vi "NHMFL SCM Oxford IPS initialize.vi"(0 "VISA session":refnum<visa-resource-name>="GPIB0::22::INSTR") -> (1 "dup VISA session":refnum<visa-resource-name>, 2 "Output Cluster":T2 {"MaxLambdaCurrent [A]" format="%.2f"; "LambdaRates [A/min]" format="%.5e"; "MaxNormalCurrent [A]" format="%.2f"; "StabilitySetting [%]" format="%.2f"; "FieldCurrentRatio [T/A]" format="%.2f"; "SwitchWaitTime [s]" format="%.2f"; "SwitchHtrCurrent [mA]" format="%.2f"; "TrainRates [A/min]" format="%.5e"; "NormalRates [A/min]" format="%.5e"; "Breakpts [A]" format="%.5e"}, 3 "Mode Out":T1(ring), 4 "Programmed Field":dbl format="%.2f", 5 "Ramp Rate":dbl format="%.2f", 6 "Persistent Field":dbl format="%.2f", 7 "Persistent":bool)   [LabVIEW 2024]
panel:
  in  "Input Cluster":T2 {"MaxLambdaCurrent [A]" format="%.2f"; "LambdaRates [A/min]" format="%.5e"; "MaxNormalCurrent [A]" format="%.2f"; "StabilitySetting [%]" format="%.2f"; "FieldCurrentRatio [T/A]" format="%.2f"; "SwitchWaitTime [s]" format="%.2f"; "SwitchHtrCurrent [mA]" format="%.2f"; "TrainRates [A/min]" format="%.5e"; "NormalRates [A/min]" format="%.5e"; "Breakpts [A]" format="%.5e"}
  out "Field":dbl format="%.2f"
  out "error out":errorcluster
  in  "error in (no error)":errorcluster
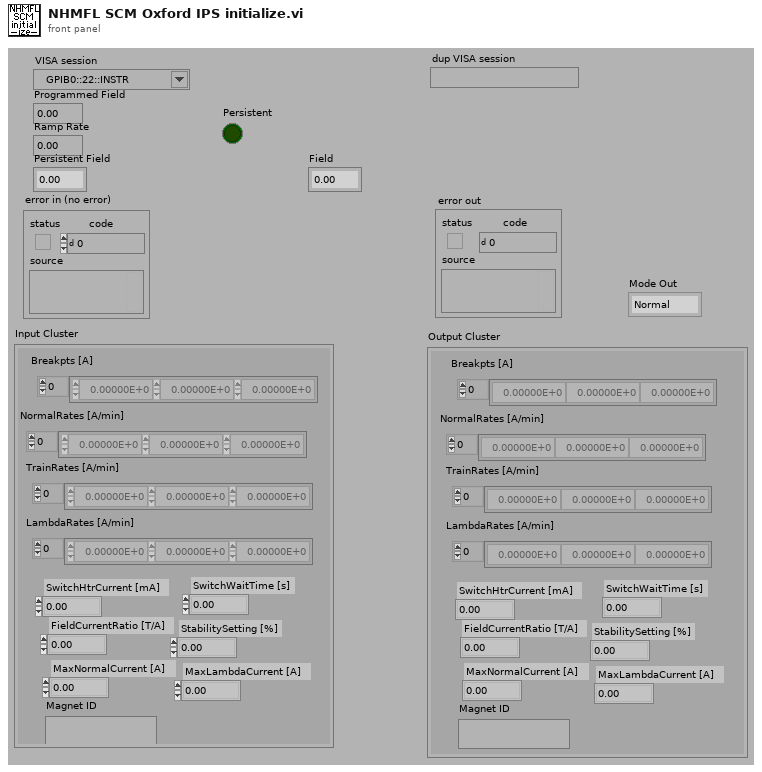
[diagram p1: front panel]
types:
  T1 = enum16{"Normal", "Train", "Lambda", "Train & Lambda"}
  T2 = cluster{"Breakpts [A]":dbl[], "NormalRates [A/min]":dbl[], "TrainRates [A/min]":dbl[], "SwitchHtrCurrent [mA]":dbl, "SwitchWaitTime [s]":dbl, "FieldCurrentRatio [T/A]":dbl, "StabilitySetting [%]":dbl, "MaxNormalCurrent [A]":dbl, "Magnet ID":string, "LambdaRates [A/min]":dbl[], "MaxLambdaCurrent [A]":dbl}
  T3 = enum16{"No Response", "Ramping to programmed field ", "Holding at programmed field", "Paused", "Ramp Manual Up", "Ramp Manual Down", "Ramping to Zero", "QUENCH", "Heating Persistence Switch", "At Zero Current"}
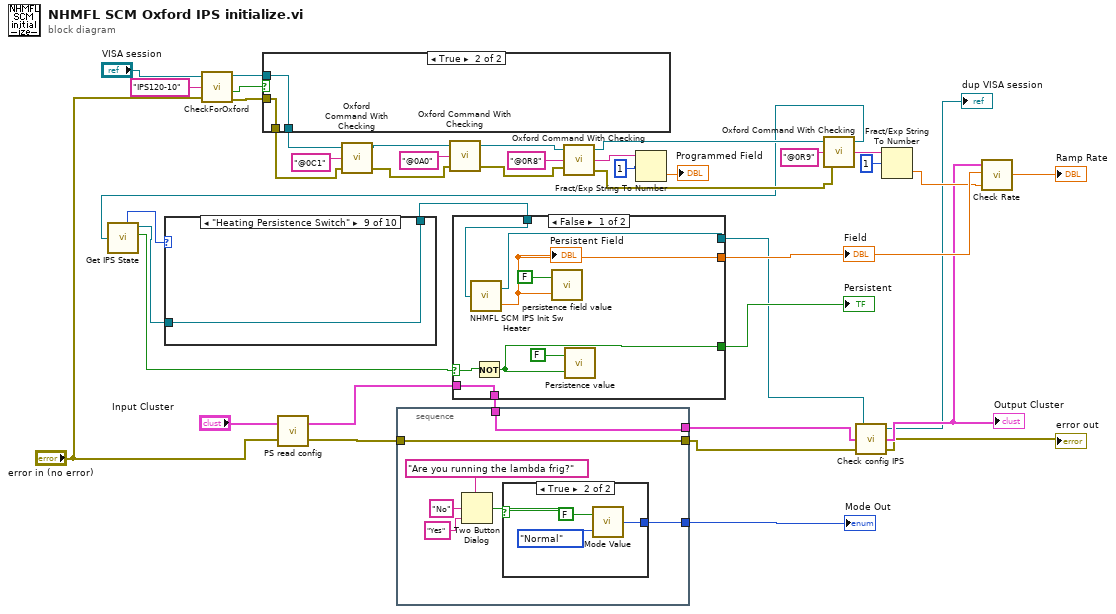
[diagram p0: block diagram]
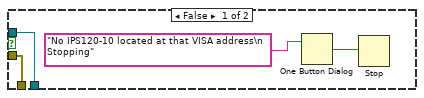
[diagram p2: hidden frame]
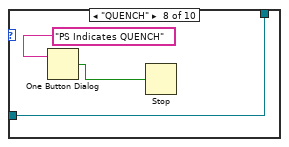
[diagram p10: hidden frame]
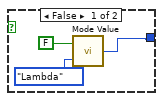
[diagram p12: hidden frame]
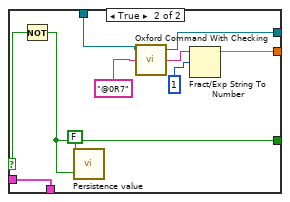
[diagram p13: hidden frame]
diagram:
  n1 = call "CheckForOxford.vi"("VISA session"="VISA session", "search string"="IPS120-10", "error in (no error)"="error in (no error)") -> ("dup VISA session"=w29:refnum<visa-resource-name>, "Instrument detected"=w31:bool, "error out"=w30:errorcluster)  [unwired: 1 out]
  n2 = case shown="True" w31 {
    tunnel: [w45 w49] -> w27
    tunnel: w30 -> [w45 w49]
    tunnel: [w44 w48] -> w16
    tunnel: w29 -> [w44 w48]
    frame False {
      n3 = One Button Dialog(message="No IPS120-10 located at that VISA address\n                                 Stopping") -> (true=w46:bool)  [unwired: 1 in]
      n4 = Stop(stop? (T)=w46) -> ()
    }
    frame True {
    }
  }
  n5 = call "PS read config.vi"("error in (no error)"="error in (no error)", "Input Cluster"="Input Cluster") -> ("error out"=w39:errorcluster, "output cluster"=w38:T2)
  n6 = call "Oxford Command With Checking.vi"("error in (no error)"=w27, "Command"="@0C1" ("Command String"), "VISA session"=w16) -> ("error out"=w7:errorcluster, "dup VISA session"=w8:refnum<visa-resource-name>)  [unwired: 1 out]
  n7 = call "Oxford Command With Checking.vi"("error in (no error)"=w7, "Command"="@0A0" ("Command String"), "VISA session"=w8) -> ("error out"=w6:errorcluster, "dup VISA session"=w5:refnum<visa-resource-name>)  [unwired: 1 out]
  n8 = call "Oxford Command With Checking.vi"("error in (no error)"=w6, "Command"="@0R8" ("Command String"), "VISA session"=w5) -> ("error out"=w19:errorcluster, "String Read"=w26:string, "dup VISA session"=w25:refnum<visa-resource-name>)
  n9 = Fract/Exp String To Number(string=w26, offset=1) -> (number=→"Programmed Field":dbl)  [unwired: 2 in, 1 out]
  n10 = call "Oxford Command With Checking.vi"("error in (no error)"=w19, "Command"="@0R9" ("Command String"), "VISA session"=w25) -> ("String Read"=w23:string, "dup VISA session"=w1:refnum<visa-resource-name>)  [unwired: 1 out]
  n11 = call "Get IPS State.vi"("VISA session"=w1) -> ("State"=w18:T3, "dup VISA session"=w3:refnum<visa-resource-name>, "Switch Heater"=w17:bool)  [unwired: 1 in, 2 out]
  n12 = case shown="\"Heating Persistence Switch\"" w18 {
    tunnel: [w50 w51 w52 w53 w54 w55 w56 w57 w60 w61] -> w35
    tunnel: w3 -> [w50 w51 w52 w53 w54 w55 w56 w57 w60 w61]
    frame "No Response", Default {
    }
    frame "Holding at programmed field" {
    }
    frame "Ramping to programmed field " {
    }
    frame "Paused" {
    }
    frame "Ramp Manual Up" {
    }
    frame "Ramp Manual Down" {
    }
    frame "Ramping to Zero" {
    }
    frame "QUENCH" {
      n13 = One Button Dialog(message="PS Indicates QUENCH") -> (true=w58:bool)  [unwired: 1 in]
      n14 = Stop(stop? (T)=w58) -> ()
    }
    frame "Heating Persistence Switch" {
    }
    frame "At Zero Current" {
    }
  }
  n15 = case shown="False" w17 {
    selector: w17 -> [w67 w78]
    tunnel: [w66 w77] -> w43
    tunnel: w35 -> [w64 w74]
    tunnel: [w63 w76] -> w40
    tunnel: w38 -> [w65 w75]
    tunnel: [w65 w75] -> w37
    tunnel: [w62 w73] -> w11
    frame False {
      n16 = call "NHMFL SCM IPS Init Sw Heater.vi"("VISA session"=w64) -> ("dup VISA session"=w62:refnum<visa-resource-name>, "Persistent Field"=w63:dbl)
      "Persistent Field" <- w63
      n17 = Not(x=w67) -> (.not. x?=w66:bool)
      n18 = call "persistence field value.vi"("Persistent Field In"=w63, "Read/Write this vi"=FALSE) -> ()  [unwired: 1 out]
      n19 = call "Persistence value.vi"("Persistence In"=w66, "Read/Write this vi"=FALSE) -> ()  [unwired: 1 out]
    }
    frame True {
      n20 = Not(x=w78) -> (.not. x?=w77:bool)
      n21 = call "Persistence value.vi"("Persistence In"=w77, "Read/Write this vi"=FALSE) -> ()  [unwired: 1 out]
      n22 = call "Oxford Command With Checking.vi"("Command"="@0R7" ("Command String"), "VISA session"=w74) -> ("String Read"=w72:string, "dup VISA session"=w73:refnum<visa-resource-name>)  [unwired: 1 in, 1 out]
      n23 = Fract/Exp String To Number(string=w72, offset=1 ("index")) -> (number=w76:dbl)  [unwired: 2 in, 1 out]
    }
  }
  "Persistent" <- w43
  "Field" <- w40
  n24 = stacked-sequence {
    tunnel: w39 -> [w82]
    tunnel: [w82] -> w13
    tunnel: [w81] -> w12
    tunnel: w37 -> [w81]
    tunnel: [w80] -> w36
    frame #0 {
      n25 = Two Button Dialog(message="Are you running the lambda frig?", 1:"Yes" ("F button name (\"Cancel\")"), 2:"No" ("T button name (\"OK\")")) -> (T button?=w83:bool)
      n26 = case shown="True" w83 {
        tunnel: [w87 w90] -> w80
        frame False {
          n27 = call "Mode Value.vi"("Mode In"=T1."Lambda", "Read/Write this vi"=FALSE) -> ("Mode Out"=w87:T1)
        }
        frame True {
          n28 = call "Mode Value.vi"("Mode In"=T1."Normal", "Read/Write this vi"=FALSE) -> ("Mode Out"=w90:T1)
        }
      }
    }
  }
  "Mode Out" <- w36
  n29 = call "Check config IPS.vi"("error in (no error)"=w13, "input cluster"=w12, "VISA session"=w11) -> ("error out"=→"error out":errorcluster, "output cluster"=w15:T2, "VISA session 2"=→"dup VISA session":refnum<visa-resource-name>)
  "Output Cluster" <- w15
  n30 = Fract/Exp String To Number(string=w23, offset=1) -> (number=w22:dbl)  [unwired: 2 in, 1 out]
  n31 = call "Check Rate.vi"("Rate"=w22, "Field"=w40, "input cluster"=w15) -> ("Checked Rate"=→"Ramp Rate":dbl)
